vi "Format DAQ Configuration Log.vi"(8 "error in (no error)":errorcluster, 11 "Instrument.Lockin in":refnum<class "Instrument.Lockin.lvclass">) -> (0 "error out":errorcluster, 1 "Array":T1[](array[typedef]), 2 "Log Paths":string, 3 "Instrument.Lockin out":refnum<class "Instrument.Lockin.lvclass">, 4 "Times":timestamp[](array[timestamp]))   [LabVIEW 2019, in "Instrument.Lockin.lvlib" / "Instrument.Lockin.lvclass"]
uses:
  Instrument.Lockin.lvclass
  Typedefs/Lockin.LogConfiguration.DAQ--Cluster.ctl
  Instrument.Lockin.lvclass/Instrument.Lockin.ctl
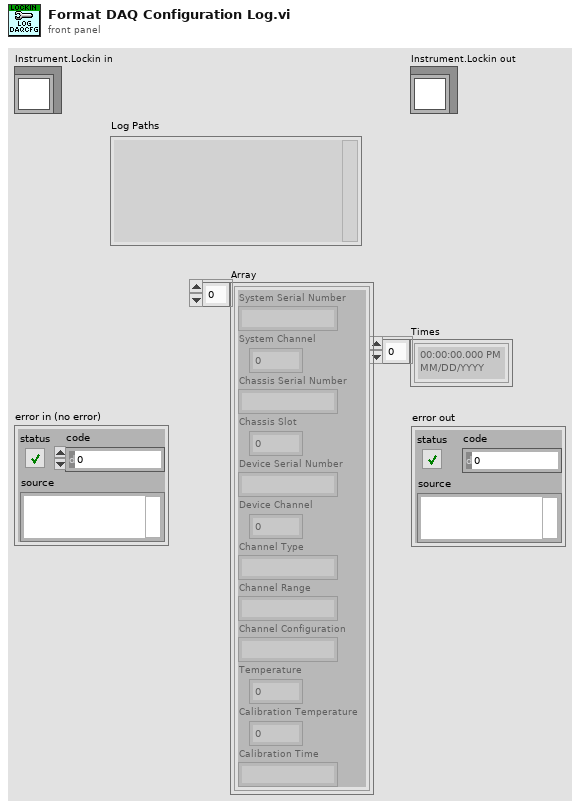
[diagram p1: front panel]
types:
  T1 = typedef "Instrument.Lockin.lvlib/Instrument.Lockin.lvclass/Lockin.LogConfiguration.DAQ--Cluster.ctl" = cluster{"System Serial Number":string, "System Channel":i32, "Chassis Serial Number":string, "Chassis Slot":i32, "Device Serial Number":string, "Device Channel":i32, "Channel Type":string, "Channel Range":string, "Channel Configuration":string, "Temperature":dbl, "Calibration Temperature":dbl, "Calibration Time":string}
  T2 = typedef "Instrument.Lockin.lvlib/Instrument.DAQ.lvclass/DeviceInfo--Cluster.ctl" = cluster{"DeviceName":string, "DevIsSimulated":bool, "DeviceSerialNumber":string, "ProductType":string, "ProductCategory":i32, "ProductNumber":u32, "ChassisNumber":u32, "SlotNumber":u32, "ChassisName":string, "ChassisSerialNumber":string, "DevTemp":dbl, "SelfCal.LastDate/Time":string, "SelfCal.LastTemp":dbl, "calibration due?":bool}
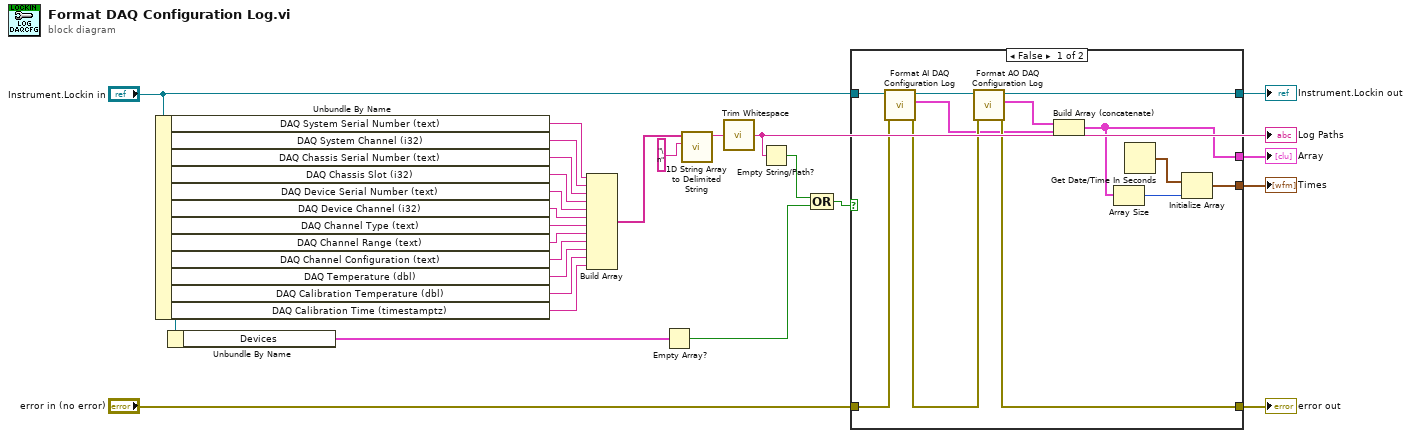
[diagram p0: block diagram]
diagram:
  n1 = Unbundle By Name("Instrument.Lockin in") -> ("DAQ System Serial Number (text)"=w21:string, "DAQ System Channel (i32)"=w20:string, "DAQ Chassis Serial Number (text)"=w19:string, "DAQ Chassis Slot (i32)"=w18:string, "DAQ Device Serial Number (text)"=w17:string, "DAQ Device Channel (i32)"=w16:string, "DAQ Channel Type (text)"=w15:string, "DAQ Channel Range (text)"=w14:string, "DAQ Channel Configuration (text)"=w13:string, "DAQ Temperature (dbl)"=w12:string, "DAQ Calibration Temperature (dbl)"=w11:string, "DAQ Calibration Time (timestamptz)"=w10:string)
  n2 = Unbundle By Name("Instrument.Lockin in") -> ("Devices"=w22:T2[])
  n3 = Build Array(w21, w20, w19, w18, w17, w16, w15, w14, w13, w12, w11, w10) -> (w9:string[])
  n4 = Empty Array?(array=w22) -> (empty?=w25:bool)
  n5 = call <vilib>:"1D String Array to Delimited String.vi"("delimiter"="\n", "string array"=w9) -> ("delimited string"=w23:string)  [unwired: 9 in]
  n6 = call <vilib>:"Trim Whitespace.vi"("string"=w23) -> ("trimmed string"=w2:string)  [unwired: 1 in]
  "Log Paths" <- w2
  n7 = Empty String/Path?(string/path=w2) -> (empty?=w8:bool)
  n8 = Compound Arithmetic op=OR(w8, w25) -> (w24:bool)
  n9 = case shown="False" w24 {
    tunnel: "error in (no error)" -> [w38 w40]
    tunnel: "Instrument.Lockin in" -> [w37 w39]
    tunnel: [w33 w40] -> w6
    tunnel: [w34 w39] -> w4
    tunnel: [w28 _] -> w3
    tunnel: [w27 _] -> w1
    frame False {
      n10 = call "Format AI DAQ Configuration Log.vi"("error in (no error)"=w38, "Instrument.Lockin in"=w37) -> ("error out"=w36:errorcluster, "Array"=w31:T1[], "Instrument.Lockin out"=w35:refnum<class "Instrument.Lockin.lvclass">)  [unwired: 7 in]
      n11 = call "Format AO DAQ Configuration Log.vi"("error in (no error)"=w36, "Instrument.Lockin in"=w35) -> ("error out"=w33:errorcluster, "Array"=w32:T1[], "Instrument.Lockin out"=w34:refnum<class "Instrument.Lockin.lvclass">)  [unwired: 7 in]
      n12 = Build Array (concatenate)(w32, w31) -> (w27:T1[])
      n13 = Array Size(array=w27) -> (size(s)=w30:i32)
      n14 = Get Date/Time In Seconds() -> (seconds since 1Jan1904=w29:timestamp)
      n15 = Initialize Array(w29, w30) -> (w28:timestamp[])
    }
    frame True {
    }
  }
  "Times" <- w3
  "error out" <- w6
  "Instrument.Lockin out" <- w4
  "Array" <- w1
